vi "test-trajectory-rotation.vi"() -> ()   [LabVIEW 2019]
uses:
  <vilib>/Rock Robotics/WPI/ThirdParty/JAS_Junk/TrajLib/TRAJ_STATE.ctl
  <vilib>/Rock Robotics/WPI/ThirdParty/JAS_Junk/TrajLib/POSE2D.ctl
  <vilib>/Rock Robotics/WPI/ThirdParty/JAS_Junk/TrajLib/TRANSLATION2D.ctl
  <vilib>/Rock Robotics/WPI/ThirdParty/JAS_Junk/TrajLib/ROTATION2D.ctl
  Robot Global Data.vi
  <vilib>/Rock Robotics/WPI/Joystick/WPI_JoystickDeviceEnum.ctl
  <vilib>/Rock Robotics/WPI/ThirdParty/JAS_Junk/TrajLib/Trajectory_Library.lvlib
panel:
  in  "Reverse":bool
  in  "Orientation \nFollows\nTravel":bool
  out "OutputTRAJ_STATE":T1={"TimeSeconds"=0.0, "Velocity"=0.0, "Acceleration"=0.0, "POSE"={"TRANSLATION"={"X"=0.0, "Y"=0.0}, "ROTATION"={"VALUE"=0.0, "COS"=1.0, "SIN"=0.0}}, "Curvature"=0.0} {"POSE"."ROTATION"."SIN" format="%13.4f"; "POSE"."ROTATION"."COS" format="%13.4f"; "POSE"."ROTATION"."VALUE" format="%13.4f"; "POSE"."TRANSLATION"."Y" format="%14.3f"; "POSE"."TRANSLATION"."X" format="%14.3f"}
  in  "Rel  Traj Time":dbl step=0.1
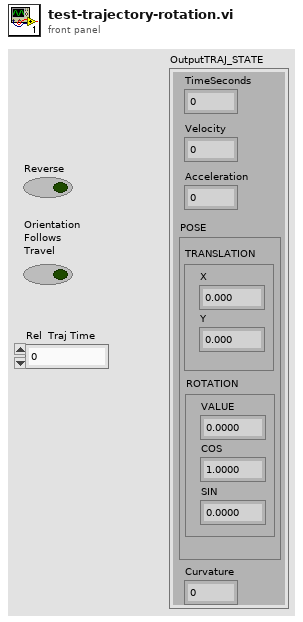
[diagram p1: front panel]
types:
  T1 = typedef "Trajectory_Library.lvlib/TRAJ_STATE.ctl" = cluster{"TimeSeconds":dbl, "Velocity":dbl, "Acceleration":dbl, "POSE":T2, "Curvature":dbl}
  T2 = typedef "Trajectory_Library.lvlib/POSE2D.ctl" = cluster{"TRANSLATION":T3, "ROTATION":T4}
  T3 = typedef "Trajectory_Library.lvlib/TRANSLATION2D.ctl" = cluster{"X":dbl, "Y":dbl}
  T4 = typedef "Trajectory_Library.lvlib/ROTATION2D.ctl" = cluster{"VALUE":dbl, "COS":dbl, "SIN":dbl}
  T5 = typedef "WPI_JoystickDeviceEnum.ctl" = enum16{"USB 0", "USB 1", "USB 2", "USB 3", "USB 4", "USB 5"}
  T6 = typedef "WPI_JoystickDevRef.ctl" = cluster{"Device":T5}
  T7 = typedef "Trajectory_Library.lvlib/TRAJECTORY.ctl" = cluster{"TotalTImeSecs":dbl, "States":T1[]}
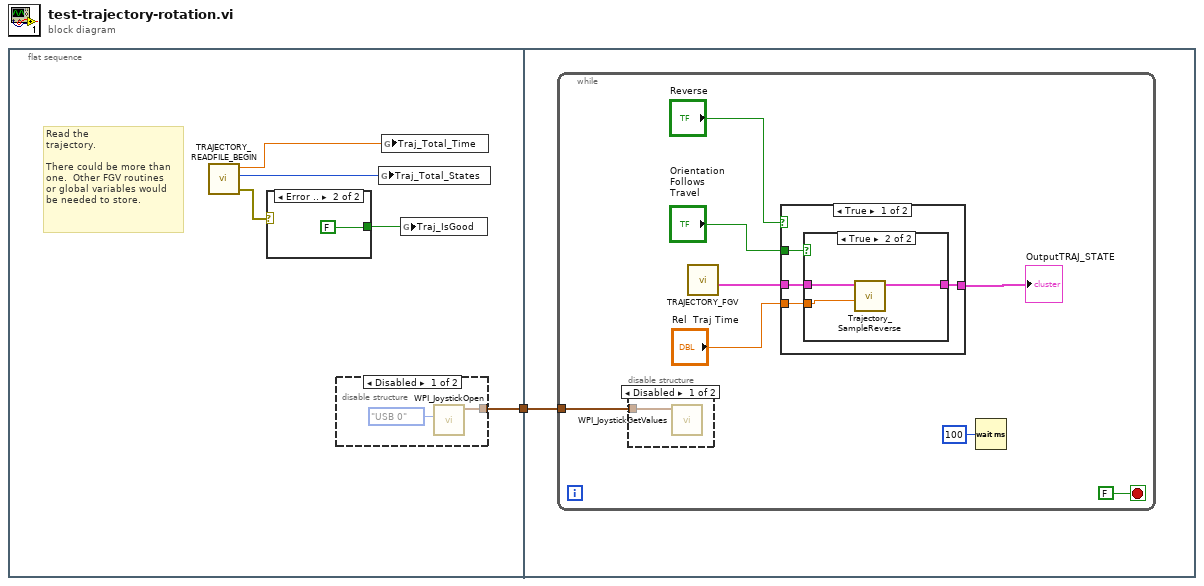
[diagram p0: block diagram]
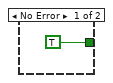
[diagram p3: hidden frame]
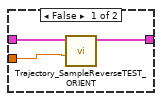
[diagram p5: hidden frame]
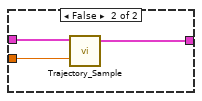
[diagram p6: hidden frame]
diagram:
  n1 = flat-sequence {
    tunnel: [w2] -> w1
    tunnel: w1 -> [w11]
    frame #0 {
      # "Read the\ntrajectory.\n\nThere could be more than\none.  Other FGV routines\nor global variables would\nbe needed to store."
      n2 = call "TRAJECTORY_READFILE_BEGIN.vi"() -> ("error out"=w6:errorcluster, "Trajectory Items"=w3:i32, "TotalTImeSecs"=w4:dbl)  [unwired: 9 in]
      n3 = case shown="Error .." w6 {
        tunnel: [TRUE FALSE] -> w5
        frame No Error {
        }
        frame Error {
        }
      }
      n4 = disable-structure shown="Disabled" {
        disable-tunnel: [w8 _] -> w2
        frame Disabled {
          n5 = call <vilib>:"WPI_JoystickOpen.vi"("JoystickDevice"=WPI_JoystickDeviceEnum."USB 0") -> ("JoystickDevRef"=w8:T6)  [unwired: 10 in]
        }
        frame Enabled {
        }
      }
      n6 = global write "Robot Global Data.vi" "Traj_Total_States"(w3) -> ()
      n7 = global write "Robot Global Data.vi" "Traj_Total_Time"(w4) -> ()
      n8 = global write "Robot Global Data.vi" "Traj_IsGood"(w5) -> ()
    }
    frame #1 {
      n9 = while {
        tunnel: w11 -> [w19]
        stop <- FALSE stop-if-true
        n10 = disable-structure shown="Disabled" {
          disable-tunnel: w19 -> [w20 _]
          frame Disabled {
            n11 = call <vilib>:"WPI_JoystickGetValues.vi"("JoystickDevRef"=w20) -> ()  [unwired: 6 in, 5 out]
          }
          frame Enabled {
          }
        }
        n12 = call "TRAJECTORY_FGV.vi"() -> ("outTRAJECTORY"=w18:T7)  [unwired: 11 in]
        n13 = case shown="True" "Reverse" {
          tunnel: w18 -> [w24 w33]
          tunnel: "Rel  Traj Time" -> [w22 w32]
          tunnel: [w23 w31] -> w16
          tunnel: "Orientation \nFollows\nTravel" -> [w21 _]
          frame True {
            n14 = case shown="True" w21 {
              tunnel: w24 -> [w27 w30]
              tunnel: [w26 w29] -> w23
              tunnel: w22 -> [w25 w28]
              frame False {
                n15 = call "Trajectory_SampleReverseTEST_ORIENT.vi"("Time"=w25, "InputTRAJECTORY"=w27) -> ("OutputTRAJ_STATE"=w26:T1)  [unwired: 9 in]
              }
              frame True {
                n16 = call <vilib>:"Trajectory_SampleReverse.vi"("Time"=w28, "InputTRAJECTORY"=w30) -> ("OutputTRAJ_STATE"=w29:T1)  [unwired: 9 in]
              }
            }
          }
          frame False {
            n17 = call <vilib>:"Trajectory_Sample.vi"("Time"=w32, "InputTRAJECTORY"=w33) -> ("OutputTRAJ_STATE"=w31:T1)  [unwired: 9 in]
          }
        }
        "OutputTRAJ_STATE" <- w16
        n18 = Wait (ms)(milliseconds to wait=u32 100) -> ()  [unwired: 1 out]
      }
    }
  }
